vi "RT Driver VI.vi"(6 "Device Clock":string, 10 "Device Outputs FIFO":refnum<k33>, 11 "Device Reference":T1 format="%.0x") -> ()   [LabVIEW 2017, in "Chassis TimeSync Engine.lvlib"]
uses:
  Chassis TimeSync Engine.lvlib
  <vilib>/NI Veristand/Custom Device API/Custom Device Item Ref.ctl
  <vilib>/NI Veristand/Custom Device Tools/Custom Device Utility Library/Custom Device Utility Library.lvlib
  <vilib>/NI Veristand/Custom Device API/Custom Device API.lvlib
panel:
  in  "Initialization Status Notifier":refnum<notifier>
  in  "Status Notifier":refnum<notifier>
  # "Custom Device Template\nv1.0"
  # "Use this template as a starting point for creating a custom device code module. The input controls shown here are specially named controls that the system will use to provide the device loop with data. The controls are not required for the device loop to run. For instance, if the device doesn't produce any output data, then you don't need the Device Outputs FIFO control. If you do use these controls, however, they need to have these exact names to be functional."
  # "The optional status notifier element is used to notify the RT engine of the last state of the custom device, and to indicate the device has completed execution. If this control is not used, a default No Error value is returned to the system when the device finishes execution.\n\nNote: This error state is not checked until the system shuts down. Use an output status channel to send more immediate status values to the system."
  # "This optional input can be used to send the VeriStand Engine the final status of the custom device initalization process. If this control exists on the custom device front panel, the VeriStand Engine will wait for a status update before starting up. If the custom device reports an error, that will abort the execution of the current configuration in the VeriStand Engine.\n\nThis control can be deleted if the custom device does not need to send the initialization status update."
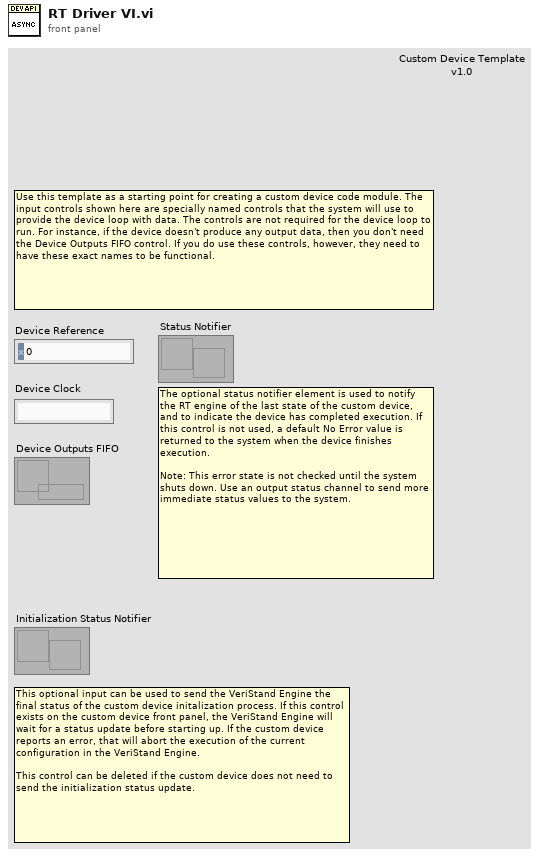
[diagram p1: front panel]
types:
  T1 = typedef "Custom Device API.lvlib/Custom Device Item Ref.ctl" = u64
  T2 = typedef "Chassis TimeSync Engine.lvlib/RT Data Cluster.ctl" = cluster{"Timekeeper hdl":refnum<k15>, "clkDisc session":T3, "Compiled Data":T4, "OutputsData":dbl[], "OutputsFIFO":refnum<k33>, "Scan Period":u32, "Timekeeper type":T14, "SyncMod type":T14, "SyncMod hdl":refnum<k15>}
  T3 = typedef "_clkDisc_session.ctl" = variant
  T4 = typedef "Chassis TimeSync Shared.lvlib/Compiled Data.ctl" = cluster{"SyncMod?":bool, "SyncMod":string, "ConnectionSettings":T5, "TimeKeeper":string, "ScanOffset(%)":dbl, "StartDelay(s)":u16, "Time Ref Settings":T10, "FIFO Locations":cluster{"SysTime":i32[], "TimeRef":i32[], "Status":i32[]}, "Clock and Trigger Routing":T13}
  T5 = typedef "Chassis TimeSync Shared.lvlib/Connection Settings.ctl" = cluster{"Mode":T6, "pxitrig":bool, "pfi0":bool, "pfi1":bool, "pfi2":bool, "External Pin":T7, "Routes":T8, "pxitrig1_ts":bool}
  T6 = typedef "Chassis TimeSync Shared.lvlib/Mode.ctl" = enum16{"Generate sample clock", "Route sample clock out of chassis", "Route sample clock into chassis", "Custom routes"}
  T7 = typedef "Chassis TimeSync Shared.lvlib/External Pin.ctl" = enum16{"PFI0", "PFI1", "PFI2"}
  T8 = typedef "Chassis TimeSync Shared.lvlib/Routes.ctl" = T9[]
  T9 = typedef "Chassis TimeSync Shared.lvlib/Route.ctl" = cluster{"Source":string, "Destination":string}
  T10 = typedef "Chassis TimeSync Shared.lvlib/Time Ref Settings.ctl" = cluster{"Time Reference":T11, "Priority 1":i32, "Priority 2":i32, "IRIG type":T12, "Terminal":string, "PPSSetTime":bool, "Start Time":timestamp}
  T11 = typedef "Chassis TimeSync Shared.lvlib/Time Reference.ctl" = enum16{"GPS", "IRIG", "PPS", "1588 Ordinary Clock", "PXI Chassis Clock", "Free Running (Internal)"}
  T12 = typedef "Chassis TimeSync Shared.lvlib/IRIG Type.ctl" = enum16{"IRIGB DC", "IRIGB AM"}
  T13 = typedef "Chassis TimeSync System Explorer.lvlib/ClockTrigger_routing.ctl" = cluster{"Shared Trigger Source Terminal (Master Chassis)":string, "Master Trigger Output":string, "Export Clock":bool, "Export Trigger":bool}
  T14 = typedef "Chassis TimeSync Engine.lvlib/timekeeper type.ctl" = enum16{"6683", "6683H", "6682", "6682H", "non-timekeeper", "timekeeper"}
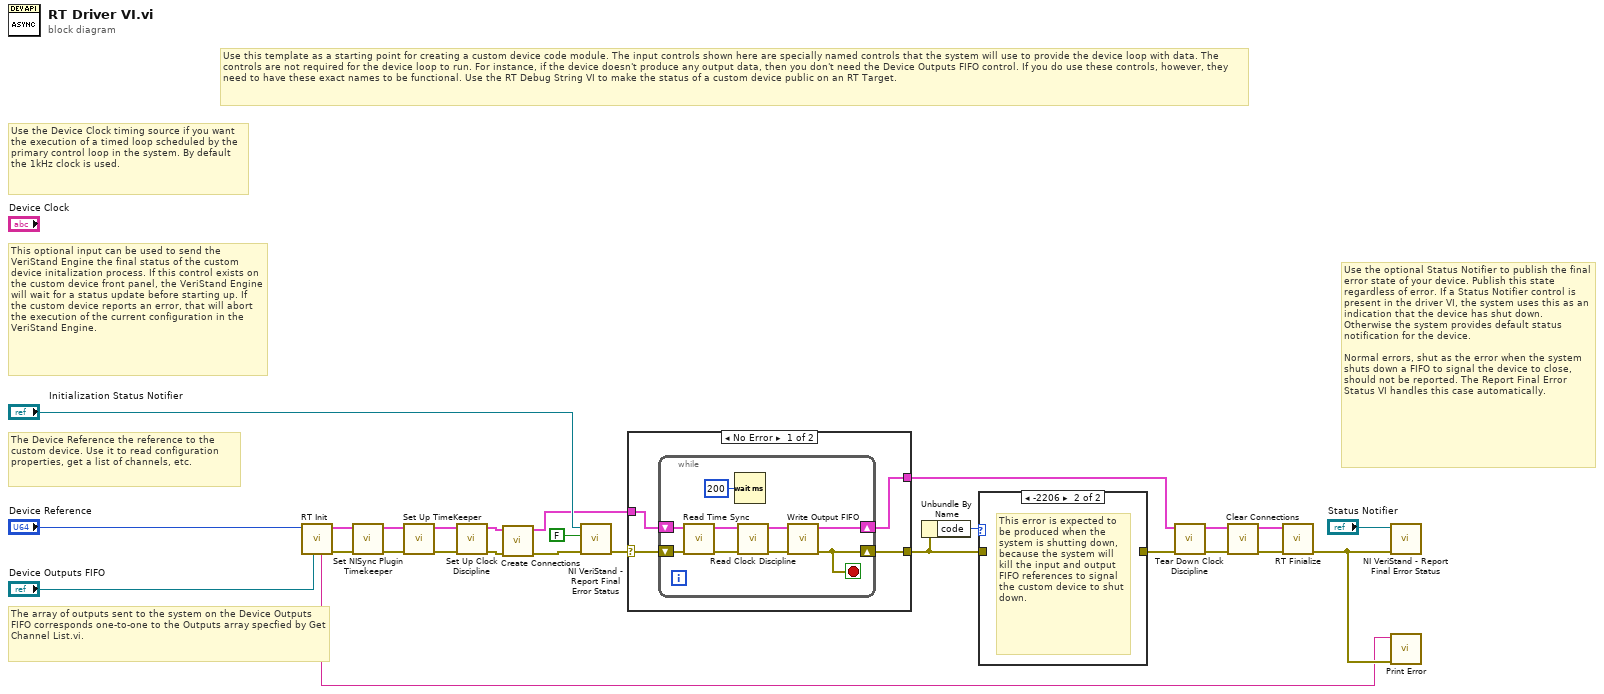
[diagram p0: block diagram]
diagram:
  # "This optional input can be used to send the VeriStand Engine the final status of the custom device initalization process. If this control exists on the custom device front panel, the VeriStand Engine will wait for a status update before starting up. If the custom device reports an error, that will abort the execution of the current configuration in the VeriStand Engine."
  # "Use the optional Status Notifier to publish the final error state of your device. Publish this state regardless of error. If a Status Notifier control is present in the driver VI, the system uses this as an indication that the device has shut down. Otherwise the system provides default status notification for the device.\n\nNormal errors, shut as the error when the system shuts down a FIFO to signal the device to close, should not be reported. The Report Final Error Status VI handles this case automatically."
  # "The array of outputs sent to the system on the Device Outputs FIFO corresponds one-to-one to the Outputs array specfied by Get Channel List.vi."
  # "The Device Reference the reference to the custom device. Use it to read configuration properties, get a list of channels, etc."
  # "Use the Device Clock timing source if you want the execution of a timed loop scheduled by the primary control loop in the system. By default the 1kHz clock is used."
  # "Use this template as a starting point for creating a custom device code module. The input controls shown here are specially named controls that the system will use to provide the device loop with data. The controls are not required for the device loop to run. For instance, if the device doesn't produce any output data, then you don't need the Device Outputs FIFO control. If you do use these controls, however, they need to have these exact names to be functional. Use the RT Debug String VI to make the status of a custom device public on an RT Target."
  n1 = call "RT Init.vi"("Device Outputs FIFO"="Device Outputs FIFO", "Device Ref"="Device Reference") -> ("error out"=w18:errorcluster, "RT Data"=w2:T2, "Name"=w4:string)  [unwired: 7 in]
  n2 = call "Set NISync Plugin Timekeeper.vi"("error in (no error)"=w18, "RT Data Cluster in"=w2) -> ("error out"=w3:errorcluster, "RT Data Cluster out"=w1:T2)  [unwired: 8 in]
  n3 = call "Set Up TimeKeeper.vi"("error in (no error)"=w3, "RT Data Cluster in"=w1) -> ("error out"=w16:errorcluster, "RT Data Cluster dup"=w15:T2)  [unwired: 8 in]
  n4 = call "Set Up Clock Discipline.vi"("error in (no error)"=w16, "RT Data Cluster in"=w15) -> ("error out"=w17:errorcluster, "RT Data Cluster out"=w9:T2)  [unwired: 8 in]
  n5 = call "Create Connections.vi"("error in (no error)"=w17, "RT Data Cluster in"=w9) -> ("error out"=w10:errorcluster, "RT Data Cluster out"=w8:T2)  [unwired: 8 in]
  n6 = call <vilib>:"NI VeriStand - Report Final Error Status.vi"("error in (no error)"=w10, "Filter FIFO & Shutdown Errors (T)"=FALSE ("Filter FIFO Errors (T)"), "Status Notifier"="Initialization Status Notifier") -> ("error out"=w23:errorcluster)  [unwired: 8 out]
  n7 = case shown="No Error" w23 {
    selector: w23 -> [w30 w41]
    tunnel: [w27 w41] -> w20
    tunnel: w8 -> [w29 w40]
    tunnel: [w28 w40] -> w13
    frame No Error {
      n8 = while "Data Loop" {
        shift-right: [w31] -> w27
        shift-left: w30 -> [w39]
        shift-right: [w37] -> w28
        shift-left: w29 -> [w38]
        stop <- w31 stop-if-true
        n9 = call "Read Time Sync.vi"("error in (no error)"=w39, "RT Data Cluster in"=w38) -> ("error out"=w35:errorcluster, "RT Data Cluster out"=w33:T2)  [unwired: 7 in, 1 out]
        n10 = Wait (ms)(milliseconds to wait=u32 200) -> ()  [unwired: 1 out]
        n11 = call "Read Clock Discipline.vi"("error in (no error)"=w35, "RT Data Cluster in"=w33) -> ("error out"=w34:errorcluster, "RT Data Cluster out"=w32:T2)  [unwired: 7 in, 1 out]
        n12 = call "Write Output FIFO.vi"("error in (no error)"=w34, "RT Data Cluster in"=w32) -> ("error out"=w31:errorcluster, "RT Data Cluster out"=w37:T2)  [unwired: 8 in]
      }
    }
    frame Error {
    }
  }
  n13 = Unbundle By Name(w20) -> ("code"=w21:i32)
  n14 = case shown="-2206" w21 {
    tunnel: [w42 _] -> w14
    tunnel: w20 -> [w42 _]
    frame 0, Default {
    }
    frame -2206 {
      # "This error is expected to be produced when the system is shutting down, because the system will kill the input and output FIFO references to signal the custom device to shut down."
    }
  }
  n15 = call "Tear Down Clock Discipline.vi"("error in (no error)"=w14, "RT Data Cluster in"=w13) -> ("error out"=w12:errorcluster, "RT Data Cluster out"=w11:T2)  [unwired: 8 in]
  n16 = call "Clear Connections.vi"("error in (no error)"=w12, "RT Data Cluster in"=w11) -> ("error out"=w7:errorcluster, "RT Data Cluster out"=w6:T2)  [unwired: 8 in]
  n17 = call "RT Finialize.vi"("error in (no error)"=w7, "RT Data Cluster in"=w6) -> ("error out"=w5:errorcluster)  [unwired: 9 in]
  n18 = call <vilib>:"NI VeriStand - Report Final Error Status.vi"("error in (no error)"=w5, "Status Notifier"="Status Notifier") -> ()  [unwired: 1 in, 9 out]
  n19 = call "Print Error.vi"("error out"=w5, "Your code's public name"=w4) -> ()  [unwired: 9 in]
